vi "Get Type.vi"(11 "Data Type in":refnum<class "Data Type.lvclass">) -> (3 "Type":string)   [LabVIEW 2020, in "Data Type.lvclass"]
uses:
  <vilib>/gpm_packages/@cs/data-type-serializer/source/Data Type/Data Type.lvclass
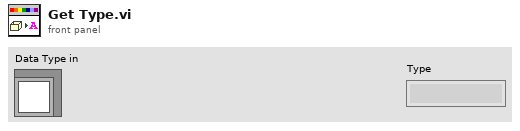
[diagram p1: front panel]
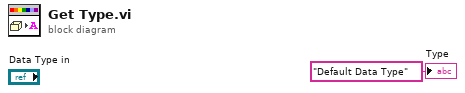
[diagram p0: block diagram]
diagram:
  "Type" <- "Default Data Type" ("Type")
